vi "value to ring (PhysErrorInjection).vi"(11 "value":string) -> (3 "PhysErrorInjection":i32(ring) items=["FDX_TX_FRAME_ERR_OFF", "FDX_TX_FRAME_ERR_CRC", "FDX_TX_FRAME_ERR_ALI", "FDX_TX_FRAME_ERR_PRE", "FDX_TX_FRAME_ERR_PHY"])   [LabVIEW 2020, in "AIM ARINC 664 Import.lvlib"]
uses:
  AIM ARINC 664 Import.lvlib
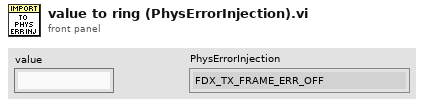
[diagram p1: front panel]
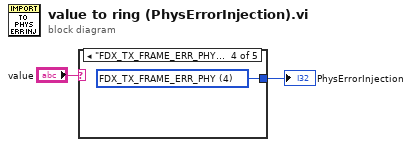
[diagram p0: block diagram]
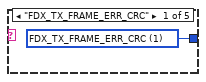
[diagram p2: hidden frame]
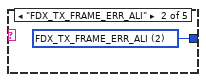
[diagram p3: hidden frame]
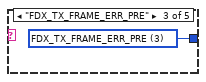
[diagram p4: hidden frame]
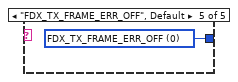
[diagram p5: hidden frame]
diagram:
  n1 = case shown="\"FDX_TX_FRAME_ERR_PHY\"" "value" {
    tunnel: [w3 w4 w5 w6 w7] -> w1
    frame "FDX_TX_FRAME_ERR_CRC" {
      w3 = 1 items=["FDX_TX_FRAME_ERR_OFF", "FDX_TX_FRAME_ERR_CRC", "FDX_TX_FRAME_ERR_ALI", "FDX_TX_FRAME_ERR_PRE", "FDX_TX_FRAME_ERR_PHY"] ("PhysErrorInjection")
    }
    frame "FDX_TX_FRAME_ERR_ALI" {
      w4 = 2 items=["FDX_TX_FRAME_ERR_OFF", "FDX_TX_FRAME_ERR_CRC", "FDX_TX_FRAME_ERR_ALI", "FDX_TX_FRAME_ERR_PRE", "FDX_TX_FRAME_ERR_PHY"] ("PhysErrorInjection")
    }
    frame "FDX_TX_FRAME_ERR_PRE" {
      w5 = 3 items=["FDX_TX_FRAME_ERR_OFF", "FDX_TX_FRAME_ERR_CRC", "FDX_TX_FRAME_ERR_ALI", "FDX_TX_FRAME_ERR_PRE", "FDX_TX_FRAME_ERR_PHY"] ("PhysErrorInjection")
    }
    frame "FDX_TX_FRAME_ERR_PHY" {
      w6 = 4 items=["FDX_TX_FRAME_ERR_OFF", "FDX_TX_FRAME_ERR_CRC", "FDX_TX_FRAME_ERR_ALI", "FDX_TX_FRAME_ERR_PRE", "FDX_TX_FRAME_ERR_PHY"] ("PhysErrorInjection")
    }
    frame "FDX_TX_FRAME_ERR_OFF", Default {
      w7 = 0 items=["FDX_TX_FRAME_ERR_OFF", "FDX_TX_FRAME_ERR_CRC", "FDX_TX_FRAME_ERR_ALI", "FDX_TX_FRAME_ERR_PRE", "FDX_TX_FRAME_ERR_PHY"] ("PhysErrorInjection")
    }
  }
  "PhysErrorInjection" <- w1
